vi "Pack_구현.vi"() -> ()   [LabVIEW 2017]
panel:
  out "*(타입 *) &x":i32
  out "부호없는 바이트 배열 2":u8[](array[numeric])
  in  "소수형 입력":dbl=3.14 format="%#_13g"
  in  "정수형 입력":i32=455000
  out "Unpack(4byte)_소수":sgl
  out "부호없는 바이트 배열":u8[](array[numeric])
  out "Pack(4byte)":string
  # "소수형 Pack(), Unpack() SW 구현"
  # "정수형 Pack(), Unpack() SW 구현"
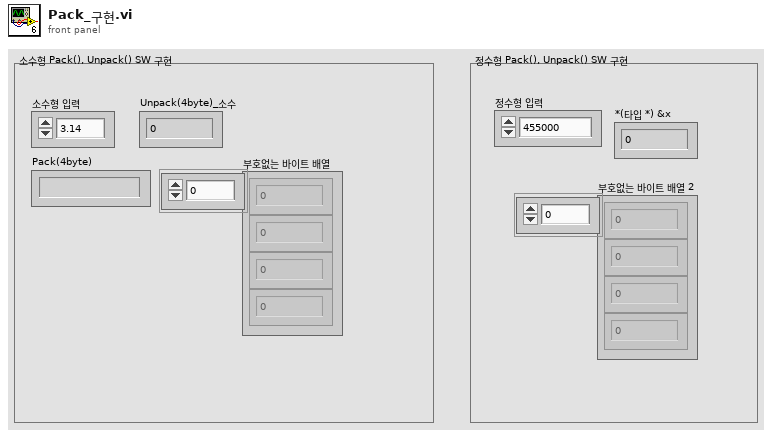
[diagram p1: front panel]
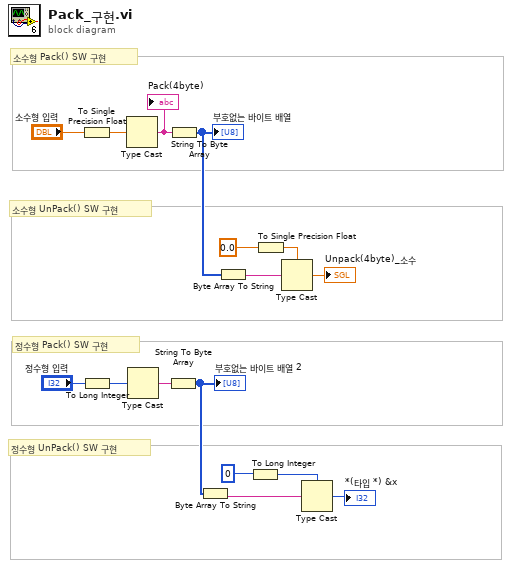
[diagram p0: block diagram]
diagram:
  # "정수형 UnPack() SW 구현"
  # "정수형 Pack() SW 구현"
  # "소수형 UnPack() SW 구현"
  # "소수형 Pack() SW 구현"
  n1 = To Single Precision Float(number="소수형 입력") -> (single precision float=w15:sgl)
  n2 = To Long Integer(number="정수형 입력") -> (32bit integer=w7:i32)
  n3 = Type Cast(x=w15) -> (*(type *) &x=w14:string)  [unwired: 1 in]
  "Pack(4byte)" <- w14
  n4 = Type Cast(x=w7) -> (*(type *) &x=w6:string)  [unwired: 1 in]
  n5 = String To Byte Array(string=w6) -> (unsigned byte array=w5:u8[])
  "부호없는 바이트 배열 2" <- w5
  n6 = String To Byte Array(string=w14) -> (unsigned byte array=w12:u8[])
  "부호없는 바이트 배열" <- w12
  n7 = Byte Array To String(unsigned byte array=w5) -> (string=w2:string)
  n8 = Byte Array To String(unsigned byte array=w12) -> (string=w11:string)
  n9 = To Long Integer(number=0 ("숫자")) -> (32bit integer=w3:i32)
  n10 = To Single Precision Float(number=0.0) -> (single precision float=w9:sgl)
  n11 = Type Cast(type=w9, x=w11) -> (*(type *) &x=→"Unpack(4byte)_소수":sgl)
  n12 = Type Cast(type=w3, x=w2) -> (*(type *) &x=→"*(타입 *) &x":i32)
